vi "Update Status Error Count.vi"(8 "unconfigured frame error":bool, 9 "error flags":T1, 10 "Values in":dbl[](array[numeric]), 11 "Rx Execution Unit Implementation in":refnum<class "Rx Execution Unit.lvclass">) -> (2 "Values out":dbl[](array[numeric]), 3 "Rx Execution Unit Implementation out":refnum<class "Rx Execution Unit.lvclass">)   [LabVIEW 2020, in "Ballard MIL-STD-1553 Engine.lvlib" / "Implementation.lvlib" / "Rx Execution Unit.lvclass"]
uses:
  Rx Execution Unit.lvclass
  <instrlib>/BTI1553Lib/Public/Controls/1553 Error Flags.ctl
  Rx Execution Unit.lvclass/Rx Execution Unit.ctl
  <instrlib>/BTI1553Lib/BTI1553LV.lvlib
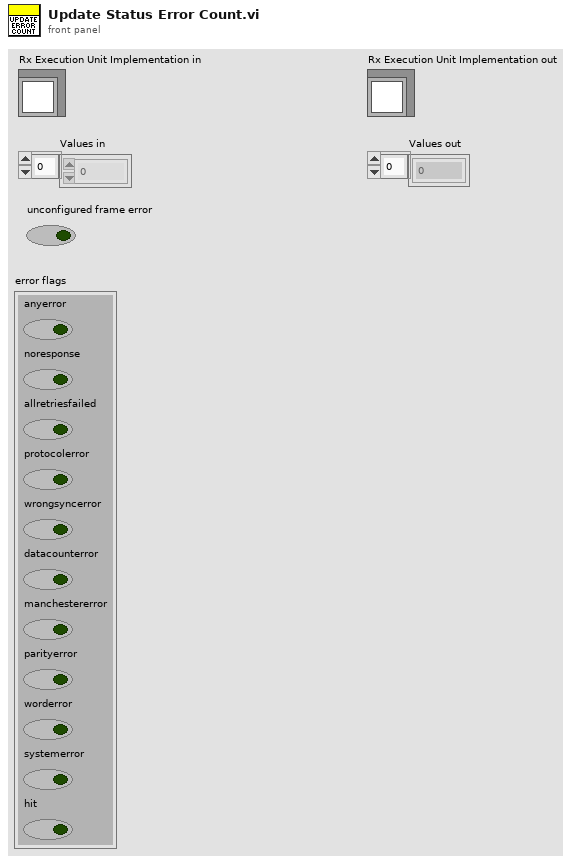
[diagram p1: front panel]
types:
  T1 = typedef "BTI1553LV.lvlib/1553 Error Flags.ctl" = cluster{"anyerror":bool, "noresponse":bool, "allretriesfailed":bool, "protocolerror":bool, "wrongsyncerror":bool, "datacounterror":bool, "manchestererror":bool, "parityerror":bool, "worderror":bool, "systemerror":bool, "hit":bool}
  T2 = typedef "Ballard MIL-STD-1553 Engine.lvlib/Implementation.lvlib/Rx Execution Unit.lvclass/Status Error Counts.ctl" = cluster{"general protocol error count":u64, "improper number of words error count":u64, "manchester error count":u64, "monitor error count":u64, "parity error count":u64, "unconfigured frames error count":u64, "word error count":u64, "wrong sync error count":u64}
  T3 = cluster{"[0]":u64, "[1]":u64, "[2]":u64, "[3]":u64, "[4]":u64, "[5]":u64, "[6]":u64, "[7]":u64}
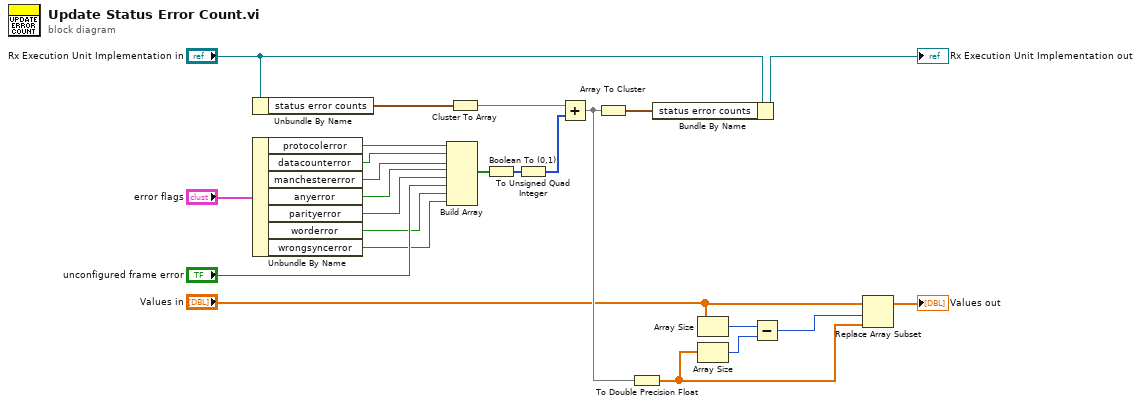
[diagram p0: block diagram]
diagram:
  n1 = Unbundle By Name("Rx Execution Unit Implementation in") -> ("status error counts"=w23:T2)
  n2 = Unbundle By Name("error flags") -> ("protocolerror"=w22:bool, "datacounterror"=w21:bool, "manchestererror"=w20:bool, "anyerror"=w19:bool, "parityerror"=w18:bool, "worderror"=w16:bool, "wrongsyncerror"=w15:bool)
  n3 = Build Array(w22, w21, w20, w19, w18, "unconfigured frame error", w16, w15) -> (w13:bool[])
  n4 = Cluster To Array(cluster=w23) -> (array=w14:u64[])
  n5 = Boolean To (0,1)(Boolean=w13) -> (0, 1=w12:i16[])
  n6 = To Unsigned Quad Integer(1:w12) -> (0:w6:u64[])
  n7 = Add(x=w14, y=w6) -> (x+y=w5:u64[])
  n8 = Array To Cluster(array=w5) -> (cluster=w11:T3)
  n9 = To Double Precision Float(number=w5) -> (double precision float=w2:dbl[])
  n10 = Bundle By Name(cluster="Rx Execution Unit Implementation in", "status error counts"=w11) -> (→"Rx Execution Unit Implementation out":refnum<class "Rx Execution Unit.lvclass">)
  n11 = Array Size(array="Values in") -> (size(s)=w8:i32)
  n12 = Array Size(array=w2) -> (size(s)=w7:i32)
  n13 = Subtract(x=w8, y=w7) -> (x-y=w3:i32)
  n14 = Replace Array Subset(array="Values in", new element=w2, index=w3) -> (→"Values out":dbl[])
